vi "sort accesses.vi"(8 "error in":errorcluster, 11 "modbus channels":refnum<class "Modbus Module Channel.lvclass">[](array[class])) -> (0 "error out":errorcluster, 3 "clump precursors":T1[](array[typedef]))   [LabVIEW 2013, in "Modbus Slave runtime.lvclass"]
uses:
  Modbus Slave runtime.lvclass
  module channel/Modbus Module Channel.lvclass
  clump precursor.ctl
  module channel/data bank type.ctl
  <vilib>/NI/Tag Bus Module Framework/channel/channel classification.ctl
  clump accesses.ctl
  <vilib>/NI/Tag Bus Module Framework/channel/TBM channel.lvclass/TBM channel.ctl
  module channel/Modbus Module Channel.lvclass/Modbus Module Channel.ctl
  <vilib>/NI/Tag Bus Module Framework/channel/Read channel classification.vi
  module channel/Read modbus type.vi
  module channel/Read starting address.vi
  <vilib>/NI/Tag Bus Module Framework/channel/TBM channel.lvclass
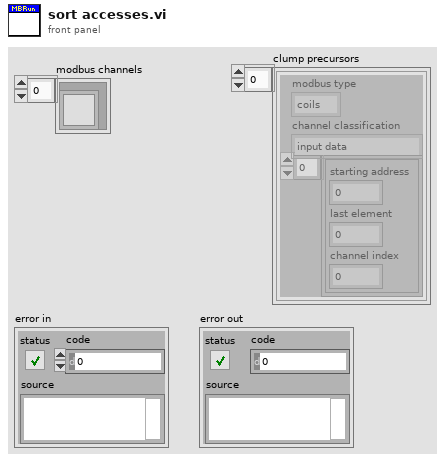
[diagram p1: front panel]
types:
  T1 = typedef "Modbus Slave runtime.lvclass/clump precursor.ctl" = cluster{"modbus type":T2, "channel classification":T3, "accesses":T4[]}
  T2 = typedef "Modbus Module Channel.lvclass/data bank type.ctl" = enum16{"coils", "discrete inputs", "input registers", "holding registers"}
  T3 = typedef "TBM channel.lvclass/channel classification.ctl" = enum16{"input data", "output data", "processing parameter", "processing result"}
  T4 = typedef "Modbus Slave runtime.lvclass/clump accesses.ctl" = cluster{"starting address":u16, "last element":i32, "channel index":i32}
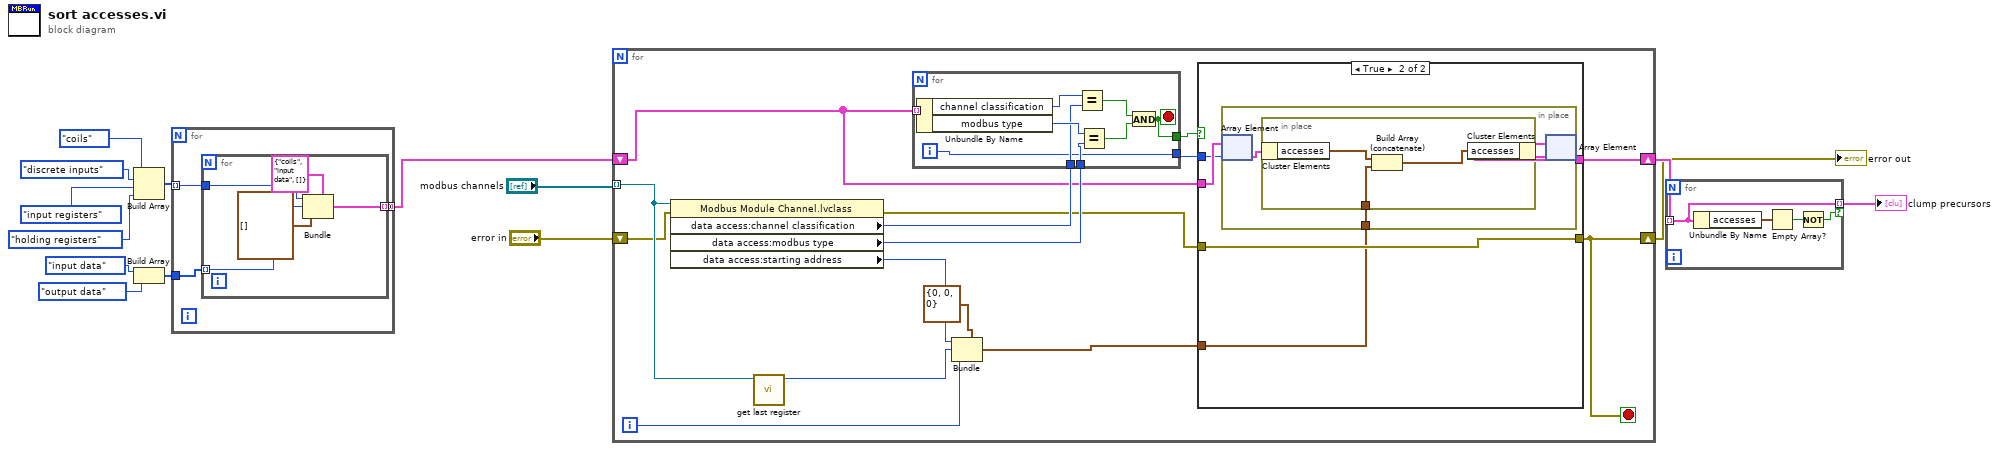
[diagram p0: block diagram]
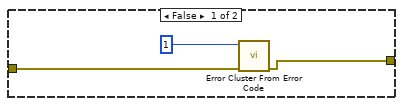
[diagram p2: hidden frame]
diagram:
  n1 = Build Array(data_bank_type."coils" ("modbus type"), data_bank_type."discrete inputs" ("modbus type"), data_bank_type."input registers" ("modbus type"), data_bank_type."holding registers" ("modbus type")) -> (w11:T2[])
  n2 = Build Array(channel_classification."input data" ("channel classification"), channel_classification."output data" ("channel classification")) -> (w12:T3[])
  n3 = for {
    tunnel: w11 -> [w17] mode=indexing
    tunnel: w12 -> [w16]
    tunnel: [w15] -> w13 mode=concatenating
    n4 = for {
      tunnel: w17 -> [w22]
      tunnel: w16 -> [w21] mode=indexing
      tunnel: [w20] -> w15 mode=indexing
      n5 = Bundle(cluster=T1 {"modbus type"=enum."coils", "channel classification"=enum."input data", "accesses"=[]} ("output cluster"), "modbus type"=w22, "channel classification"=w21, "accesses"=T4[] []) -> (w20:T1)
    }
  }
  n6 = for {
    tunnel: "modbus channels" -> [w37] mode=indexing
    shift-right: [w29] -> w2
    shift-left: w13 -> [w30]
    shift-right: [w27] -> w1
    shift-left: "error in" -> [w32]
    i -> [w23]
    stop <- w27 stop-if-true
    n7 = property class="Modbus Module Channel.lvclass"(reference=w37, error in=w32) -> (error out=w28:errorcluster, "data access:channel classification"=w34:T3, "data access:modbus type"=w33:T2, "data access:starting address"=w36:u16)  [unwired: 1 out]
    n8 = call "get last register.vi"("Modbus Module Channel in"=w37) -> ("last element"=w35:i32)  [unwired: 10 in]
    n9 = for {
      tunnel: w30 -> [w60] mode=indexing
      tunnel: w34 -> [w57]
      tunnel: w33 -> [w56]
      tunnel: [w53] -> w26
      tunnel: [w52] -> w31
      i -> [w53]
      stop <- w52 stop-if-true
      n10 = Unbundle By Name(w60) -> ("channel classification"=w58:T3, "modbus type"=w59:T2)
      n11 = Equal?(x=w58, y=w57) -> (x = y?=w54:bool)
      n12 = Equal?(x=w59, y=w56) -> (x = y?=w55:bool)
      n13 = And(x=w54, y=w55) -> (x .and. y?=w52:bool)
    }
    n14 = Bundle(cluster=T4 {"starting address"=0, "last element"=0, "channel index"=0} ("output cluster"), "starting address"=w36, "last element"=w35, "channel index"=w23) -> (w25:T4)
    n15 = case shown="True" w31 {
      tunnel: w30 -> [_ w44]
      tunnel: [_ w43] -> w29
      tunnel: [w40 w45] -> w27
      tunnel: w28 -> [w39 w45]
      tunnel: w26 -> [_ w42]
      tunnel: w25 -> [_ w41]
      frame False {
        n16 = call <vilib>:"Error Cluster From Error Code.vi"("error in (no error)"=w39, "error code (0)"=1) -> ("error out"=w40:errorcluster)  [unwired: 7 in]
      }
      frame True {
        n17 = in-place {
          in-place-border: w41 -> [w46]
          n18 = in-place-array #1(w44, w42) -> (w48:T1)
          n19 = in-place {
            in-place-border: w46 -> [w49]
            n20 = in-place-cluster #2(w48) -> ("accesses"=w51:T4[])
            n21 = Build Array (concatenate)(w51, w49) -> (w50:T4[])
            n22 = in-place-cluster #2("accesses"=w50) -> (w47:T1)
          }
          n23 = in-place-array #1(w47) -> (w43:T1[])  [unwired: 1 out]
        }
      }
    }
  }
  "error out" <- w1
  n24 = for {
    tunnel: [w64] -> w3 mode=indexing if=w62
    tunnel: w2 -> [w64] mode=indexing
    n25 = Unbundle By Name(w64) -> ("accesses"=w63:T4[])
    n26 = Empty Array?(array=w63) -> (empty?=w61:bool)
    n27 = Not(x=w61) -> (.not. x?=w62:bool)
  }
  "clump precursors" <- w3
